vi "PXI-2514 Initialization VI.vi"(8 "error in (no error)":errorcluster, 10 "Custom XML":string, 11 "Device Item Ref in":T3 format="%.0x") -> (0 "error out":errorcluster, 3 "Device Item Ref out":T3 format="%.0x")   [LabVIEW 2011, in "PXI-2514 Custom Device.lvlib"]
uses:
  PXI-2514 Custom Device.lvlib
  <vilib>/NI Veristand/Custom Device API/Custom Device Item Ref.ctl
  <vilib>/NI Veristand/Custom Device API/Custom Device Channel.ctl
  <vilib>/NI Veristand/Custom Device API/Custom Device Channel Type.ctl
  <vilib>/NI Veristand/Custom Device API/Custom Device Timed Loop Priority.ctl
  <vilib>/NI Veristand/Custom Device API/Custom Device Loop Type.ctl
  FIU Global Strings.vi
  <vilib>/NI Veristand/Custom Device API/Set Item Property (String).vi
  <vilib>/NI Veristand/Custom Device API/Set Item Property (U16).vi
  <vilib>/NI Veristand/Custom Device API/Custom Device API.lvlib
panel:
  in  "Channel":T1
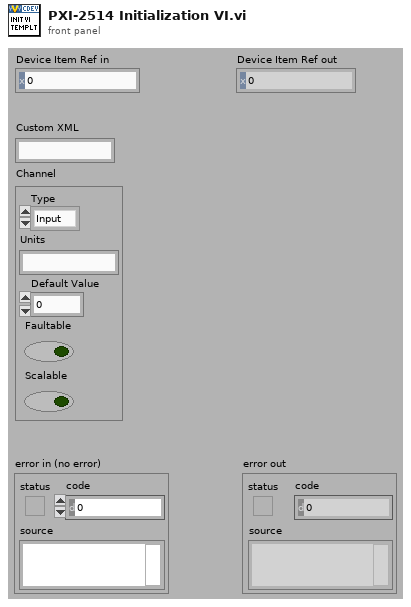
[diagram p1: front panel]
types:
  T1 = typedef "Custom Device API.lvlib/Custom Device Channel.ctl" = cluster{"Type":T2, "Units":string, "Default Value":dbl, "Faultable":bool, "Scalable":bool}
  T2 = typedef "Custom Device API.lvlib/Custom Device Channel Type.ctl" = enum16{"Input", "Output"}
  T3 = typedef "Custom Device API.lvlib/Custom Device Item Ref.ctl" = u64
  T4 = typedef "Custom Device API.lvlib/Custom Device Timed Loop Priority.ctl" = enum32{"Low", "Medium", "High"}
  T5 = typedef "Custom Device API.lvlib/Custom Device Loop Type.ctl" = enum32{"While Loop", "Timed Loop"}
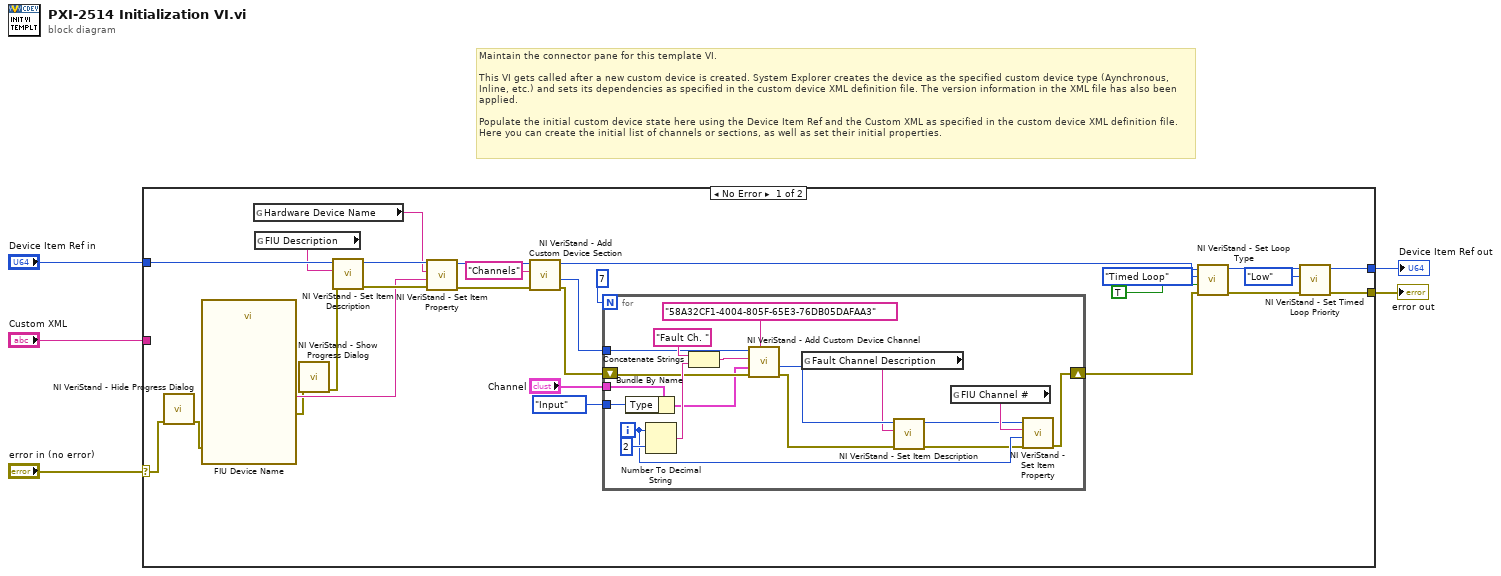
[diagram p0: block diagram]
diagram:
  # "Maintain the connector pane for this template VI.\n\nThis VI gets called after a new custom device is created. System Explorer creates the device as the specified custom device type (Aynchronous, Inline, etc.) and sets its dependencies as specified in the custom device XML definition file. The version information in the XML file has also been applied.\n\nPopulate the initial custom device state here using the Device Item Ref and the Custom XML as specified in the custom device XML definition file. Here you can create the initial list of channels or sections, as well as set their initial properties."
  n1 = case shown="No Error" "error in (no error)" {
    selector: "error in (no error)" -> [w9 w52]
    tunnel: [w13 w52] -> w5
    tunnel: [w14 w51] -> w3
    tunnel: "Device Item Ref in" -> [w32 w51]
    tunnel: "Custom XML" -> [_ _]
    frame No Error {
      n2 = call <vilib>:"NI VeriStand - Hide Progress Dialog.vi"("error in (no error)"=w9) -> ("error out"=w8:errorcluster)  [unwired: 10 in]
      n3 = call "FIU Device Name"("error in (no error)"=w8) -> ("MAX Device Name"=w12:string, "error out"=w7:errorcluster)  [unwired: 16 in, 1 out]
      n4 = global read "FIU Global Strings.vi" "Hardware Device Name"() -> (w15:string)
      n5 = global read "FIU Global Strings.vi" "FIU Description"() -> (w24:string)
      n6 = call <vilib>:"NI VeriStand - Show Progress Dialog.vi"("error in (no error)"=w7) -> ("error out"=w6:errorcluster)  [unwired: 10 in]
      n7 = call <vilib>:"NI VeriStand - Set Item Description.vi"("error in (no error)"=w6, "Description"=w24, "Item Ref in"=w32) -> ("error out"=w26:errorcluster, "Item Ref out"=w25:T3)  [unwired: 6 in, 1 out]
      n8 = call-poly <vilib>:"NI VeriStand - Set Item Property.vi"("error in (no error)"=w26, "Value"=w12, "Property Name"=w15, "Item Ref in"=w25) -> ("error out"=w22:errorcluster, "Item Ref out"=w18:T3)  [unwired: 5 in, 1 out]
      n9 = call <vilib>:"NI VeriStand - Add Custom Device Section.vi"("error in (no error)"=w22, "Section Name"="Channels", "Parent Ref in"=w18) -> ("error out"=w20:errorcluster, "Section Ptr"=w16:T3, "Parent Ref out"=w10:T3)  [unwired: 5 in, 1 out]
      n10 = for {
        N: 7 -> [_]
        tunnel: "Channel" -> [w49]
        tunnel: Custom_Device_Channel_Type."Input" ("Type") -> [w45]
        shift-right: [w38] -> w11
        shift-left: w20 -> [w44]
        tunnel: w16 -> [w42]
        i -> [w40]
        n11 = Bundle By Name(cluster=w49, "Type"=w45) -> (w43:T1)
        n12 = Number To Decimal String(number=w40, width (-)=i16 2) -> (decimal integer string=w47:string)
        n13 = Concatenate Strings("Fault Ch. " ("Section Name"), w47) -> (w46:string)
        n14 = call <vilib>:"NI VeriStand - Add Custom Device Channel.vi"("GUID (Default Channel)"="58A32CF1-4004-805F-65E3-76DB05DAFAA3", "error in (no error)"=w44, "Channel"=w43, "Channel Name"=w46, "Parent Ref in"=w42) -> ("error out"=w35:errorcluster, "Channel Ref"=w37:T3)  [unwired: 3 in, 2 out]
        n15 = global read "FIU Global Strings.vi" "Fault Channel Description"() -> (w33:string)
        n16 = call <vilib>:"NI VeriStand - Set Item Description.vi"("error in (no error)"=w35, "Description"=w33, "Item Ref in"=w37) -> ("error out"=w34:errorcluster, "Item Ref out"=w36:T3)  [unwired: 6 in, 1 out]
        n17 = global read "FIU Global Strings.vi" "FIU Channel #"() -> (w41:string)
        n18 = call-poly <vilib>:"NI VeriStand - Set Item Property.vi"("error in (no error)"=w34, "Value"=w40, "Property Name"=w41, "Item Ref in"=w36) -> ("error out"=w38:errorcluster)  [unwired: 5 in, 2 out]
      }
      n19 = call <vilib>:"NI VeriStand - Set Loop Type.vi"("error in (no error)"=w11, "Use Device Clock (Timed Loops only)"=TRUE, "Loop type"=Custom_Device_Loop_Type."Timed Loop", "Device Ref in"=w10) -> ("error out"=w27:errorcluster, "Device Ref out"=w28:T3)  [unwired: 6 in]
      n20 = call <vilib>:"NI VeriStand - Set Timed Loop Priority.vi"("error in (no error)"=w27, "Priority"=Custom_Device_Timed_Loop_Priority."Low", "Device Ref in"=w28) -> ("error out"=w13:errorcluster, "Device Ref out"=w14:T3)  [unwired: 7 in]
    }
    frame Error {
    }
  }
  "error out" <- w5
  "Device Item Ref out" <- w3
